vi "Boolean array calculations.vi"(0 "Operator":enum16{"AND", "OR"}(ring), 1 "Array1":bool[](array[boolean]), 2 "Array 2":bool[](array[boolean]), 3 "Array 3":bool[](array[boolean])) -> (14 "Array out":bool[](array[boolean]))   [LabVIEW 2020]
doc: "This VI performs a boolean operation of up to three boolean input arrays. The difference to LabVIEWs own boolean operators is that the input arrays can have different sizes. The missing elements are considered to be FALSE elements and the resulting array contains the maximum number of elements."
panel:
  # "This vi performs a boolean operation of up to three boolean input arrays. \nThe difference to LabVIEWs own boolean operators is that the input arrays\ncan have different sizes. The missing elements are considered to be FALSE\nelements and the resulting array contains the maximum number of elements."
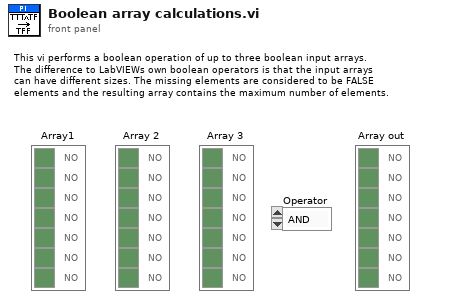
[diagram p1: front panel]
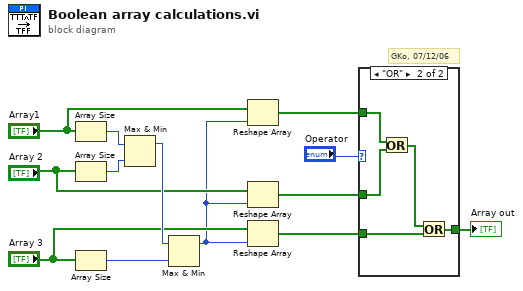
[diagram p0: block diagram]
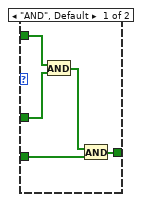
[diagram p2: hidden frame]
diagram:
  # "GKo, 07/12/06"
  n1 = Array Size(array="Array1") -> (size(s)=w13:i32)
  n2 = Array Size(array="Array 2") -> (size(s)=w12:i32)
  n3 = Array Size(array="Array 3") -> (size(s)=w10:i32)
  n4 = Max & Min(x=w13, y=w12) -> (max(x,y)=w11:i32)  [unwired: 1 out]
  n5 = Max & Min(x=w11, y=w10) -> (max(x,y)=w6:i32)  [unwired: 1 out]
  n6 = Reshape Array("Array1", w6) -> (w4:bool[])
  n7 = Reshape Array("Array 2", w6) -> (w3:bool[])
  n8 = Reshape Array("Array 3", w6) -> (w2:bool[])
  n9 = case shown="\"OR\"" "Operator" {
    tunnel: w4 -> [w18 w23]
    tunnel: w3 -> [w17 w22]
    tunnel: w2 -> [w15 w20]
    tunnel: [w14 w19] -> w1
    frame "AND", Default {
      n10 = And(x=w18, y=w17) -> (x .and. y?=w16:bool[])
      n11 = And(x=w16, y=w15) -> (x .and. y?=w14:bool[])
    }
    frame "OR" {
      n12 = Or(x=w23, y=w22) -> (x .or. y?=w21:bool[])
      n13 = Or(x=w21, y=w20) -> (x .or. y?=w19:bool[])
    }
  }
  "Array out" <- w1
